vi "GetGPIBAddress.vi"(8 "error in (no error)":errorcluster, 11 "VISA resource name":refnum<visa-resource-name>) -> (0 "error out":errorcluster, 2 "GPIB address":string, 3 "VISA resource name out":refnum<visa-resource-name>)   [LabVIEW 2016]
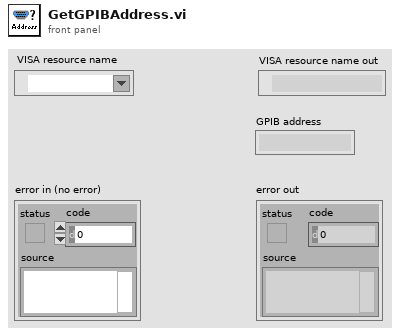
[diagram p1: front panel]
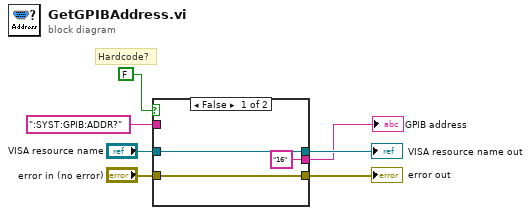
[diagram p0: block diagram]
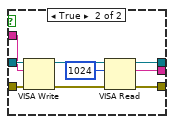
[diagram p2: hidden frame]
diagram:
  # "Hardcode?"
  n1 = case shown="False" FALSE {
    tunnel: "error in (no error)" -> [w9 w16]
    tunnel: "VISA resource name" -> [w10 w15]
    tunnel: ":SYST:GPIB:ADDR?" -> [_ w14]
    tunnel: [w10 w13] -> w4
    tunnel: [w9 w12] -> w3
    tunnel: ["16" ("read buffer") w11] -> w2
    frame False {
    }
    frame True {
      n2 = VISA Write(VISA resource name=w15, write buffer=w14, error in (no error)=w16) -> (VISA resource name out=w18:refnum<visa-resource-name>, error out=w19:errorcluster)  [unwired: 1 out]
      n3 = VISA Read(VISA resource name=w18, byte count=u32 1024, error in (no error)=w19) -> (VISA resource name out=w13:refnum<visa-resource-name>, read buffer=w11:string, error out=w12:errorcluster)  [unwired: 1 out]
    }
  }
  "error out" <- w3
  "VISA resource name out" <- w4
  "GPIB address" <- w2
